vi "2D Write.vi"(0 "Task":refnum<k21>, 1 "samples per channel":i32=1000, 2 "rate":dbl=2.0 format="%0.2f", 3 "Error In":errorcluster, 4 "data":dbl[][](array[numeric]) format="%0.2f") -> (5 "task out":refnum<k21>, 6 "Error Out":errorcluster)   [LabVIEW 2012]
doc: "Плавное изменение напряжения от старого значения до нового"
uses:
  <vilib>/DAQmx/configure/timing.llb/DAQmx Timing (Sample Clock).vi
  <vilib>/DAQmx/write.llb/DAQmx Write (Analog 2D DBL NChan NSamp).vi
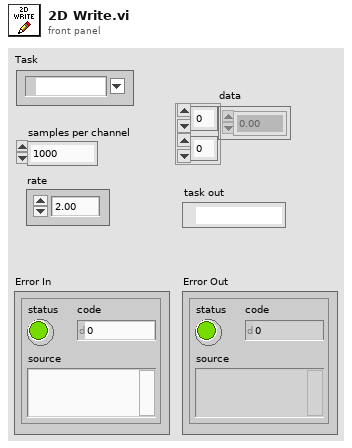
[diagram p1: front panel]
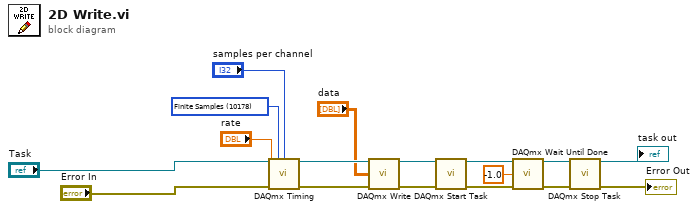
[diagram p0: block diagram]
diagram:
  w16 = 10178 items=["Finite Samples"=10178, "Continuous Samples"=10123, "Hardware Timed Single Point"=12522] ("sample mode")
  n1 = call-poly <vilib>:"DAQmx Timing.vi"("task/channels in"="Task", "sample mode"=w16, "samples per channel"="samples per channel", "rate"="rate", "error in"="Error In") -> ("task out"=w15:refnum<k21>, "error out"=w14:errorcluster)  [unwired: 9 in]
  n2 = call-poly <vilib>:"DAQmx Write.vi"("task/channels in"=w15, "data"="data", "error in"=w14) -> ("task out"=w13:refnum<k21>, "error out"=w12:errorcluster)  [unwired: 10 in, 1 out]
  n3 = call <vilib>:"DAQmx Start Task.vi"("task/channels in"=w13, "error in"=w12) -> ("task out"=w11:refnum<k21>, "error out"=w10:errorcluster)  [unwired: 12 in]
  n4 = call <vilib>:"DAQmx Wait Until Done.vi"("task/channels in"=w11, "timeout (sec)"=-1.0, "error in"=w10) -> ("task out"=w8:refnum<k21>, "error out"=w2:errorcluster)  [unwired: 11 in]
  n5 = call <vilib>:"DAQmx Stop Task.vi"("task/channels in"=w8, "error in"=w2) -> ("task out"=→"task out":refnum<k21>, "error out"=→"Error Out":errorcluster)  [unwired: 12 in]
